vi "主画面.vi"() -> ()   [LabVIEW 2016]
uses:
  <vilib>/Utility/sysdir.llb/System Directory Type.ctl
  data/FreeMem.dll
  API/update/update/update.lvlib
panel:
  out "SN":string="系列号"
  in  "关于":bool
  in  "全屏":T1
  out "站点名称":string="站点名称"
  out "时间显示":string="2017-05-09 10:50:42"
  in  "主画面菜单":enum32{"首页", "数据查询", "运维调试", "系统设置"}(xcontrol)
  # "ESTD-XP一体化水质自动监测系统"
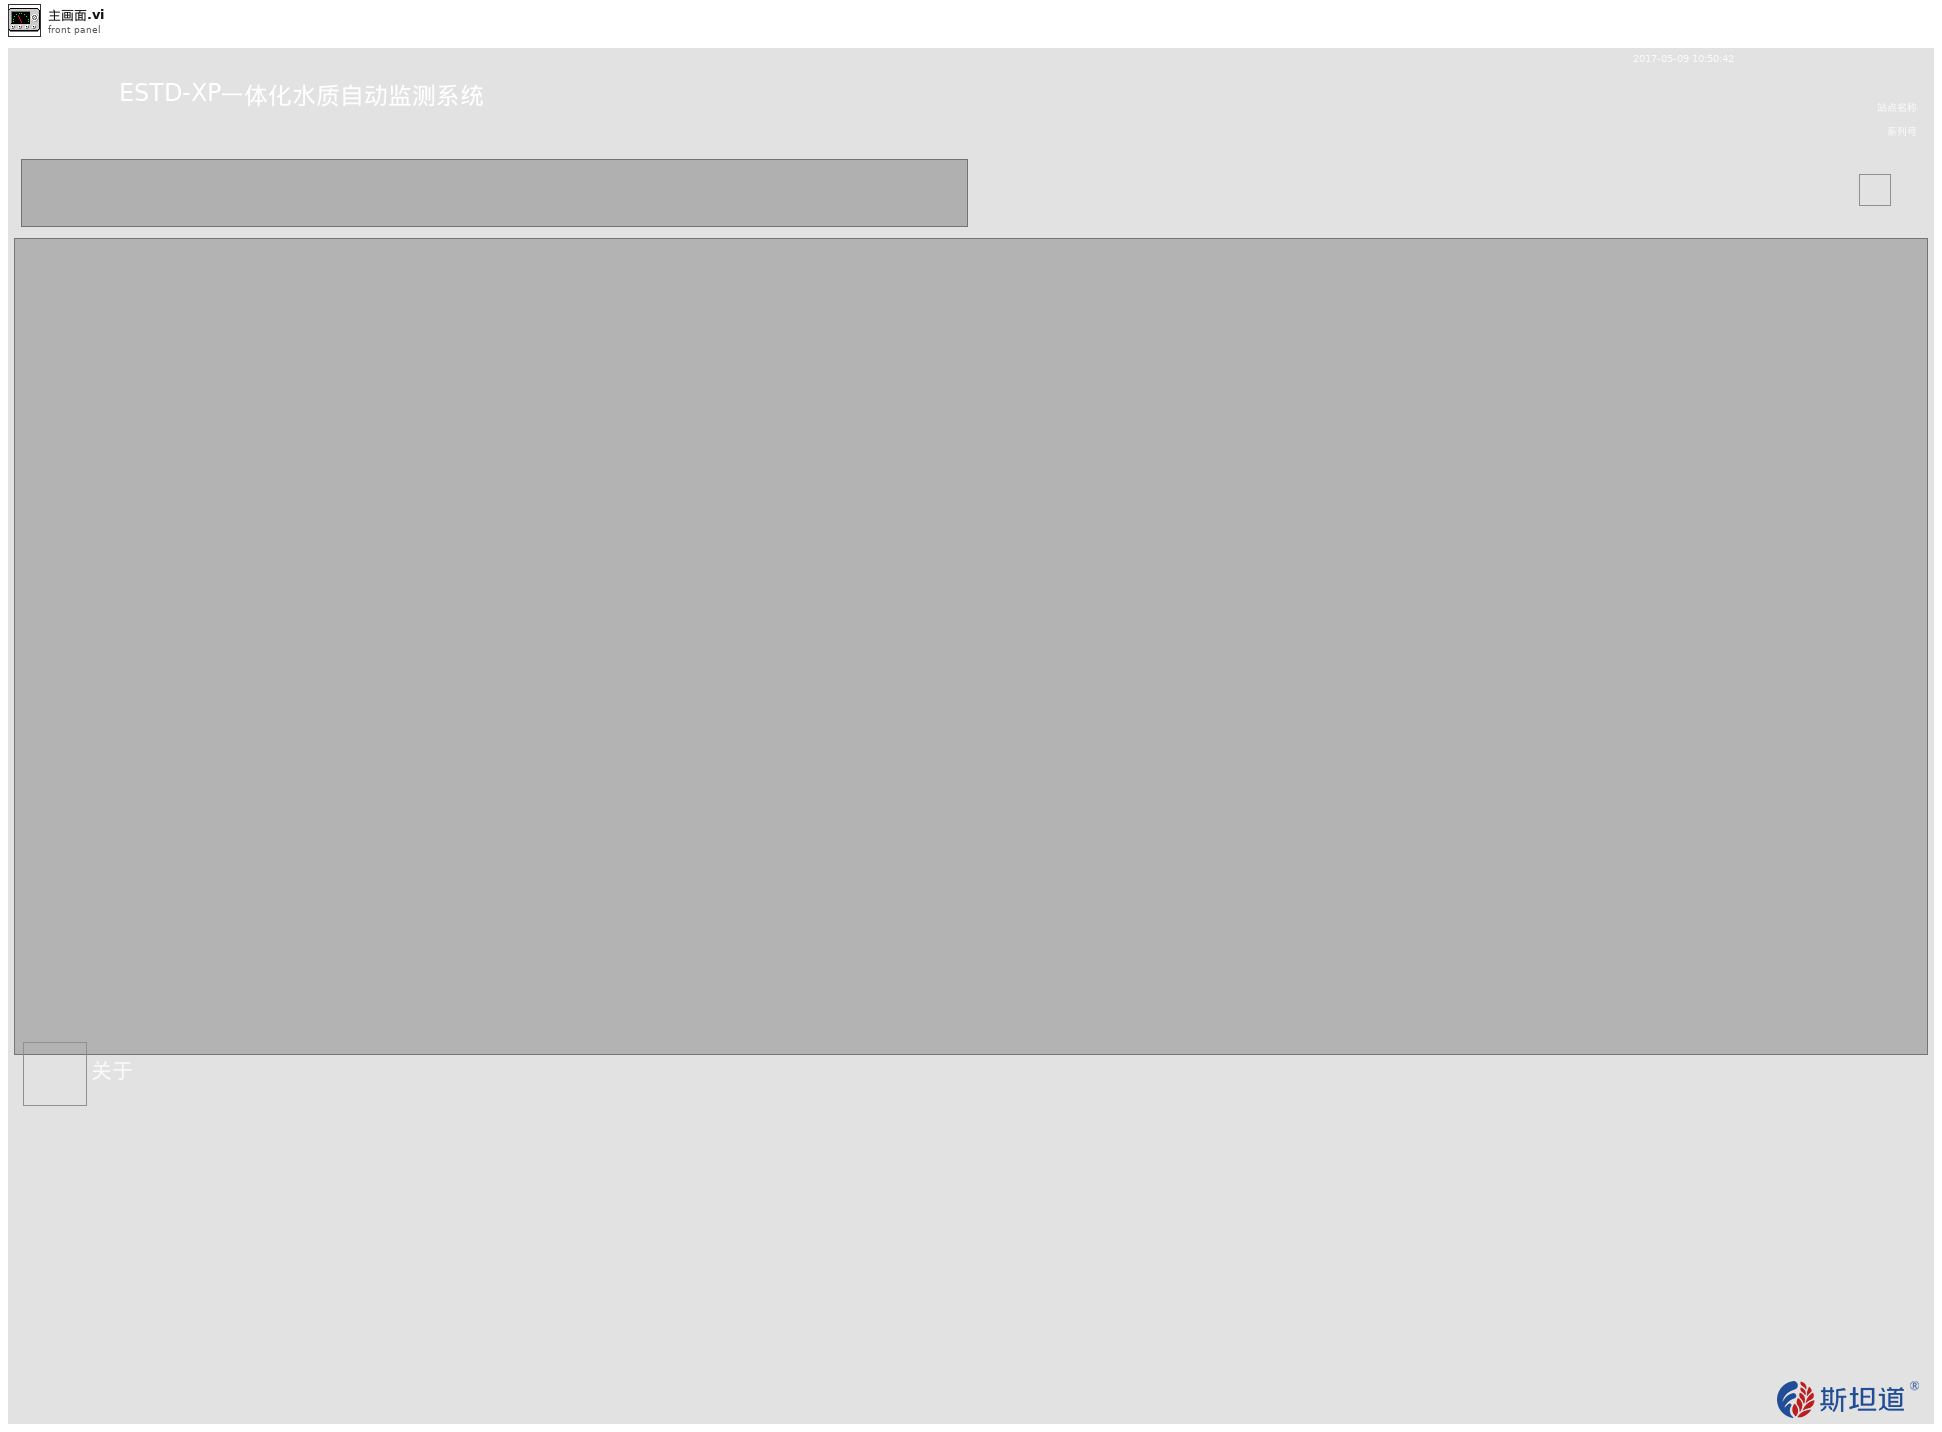
[diagram p1: front panel]
types:
  T1 = typedef "全屏按钮.ctl" = bool
  T2 = typedef "System Directory Type.ctl" = i32
  T3 = cluster{"时间标识":timestamp, "设备":string, "日志信息":string, "流程参数":string}
  T4 = enum32{"Bad", "Idle", "Run top level", "Running"}
  T5 = cluster{"host":string, "user":string, "password":string, "远端地址":string}
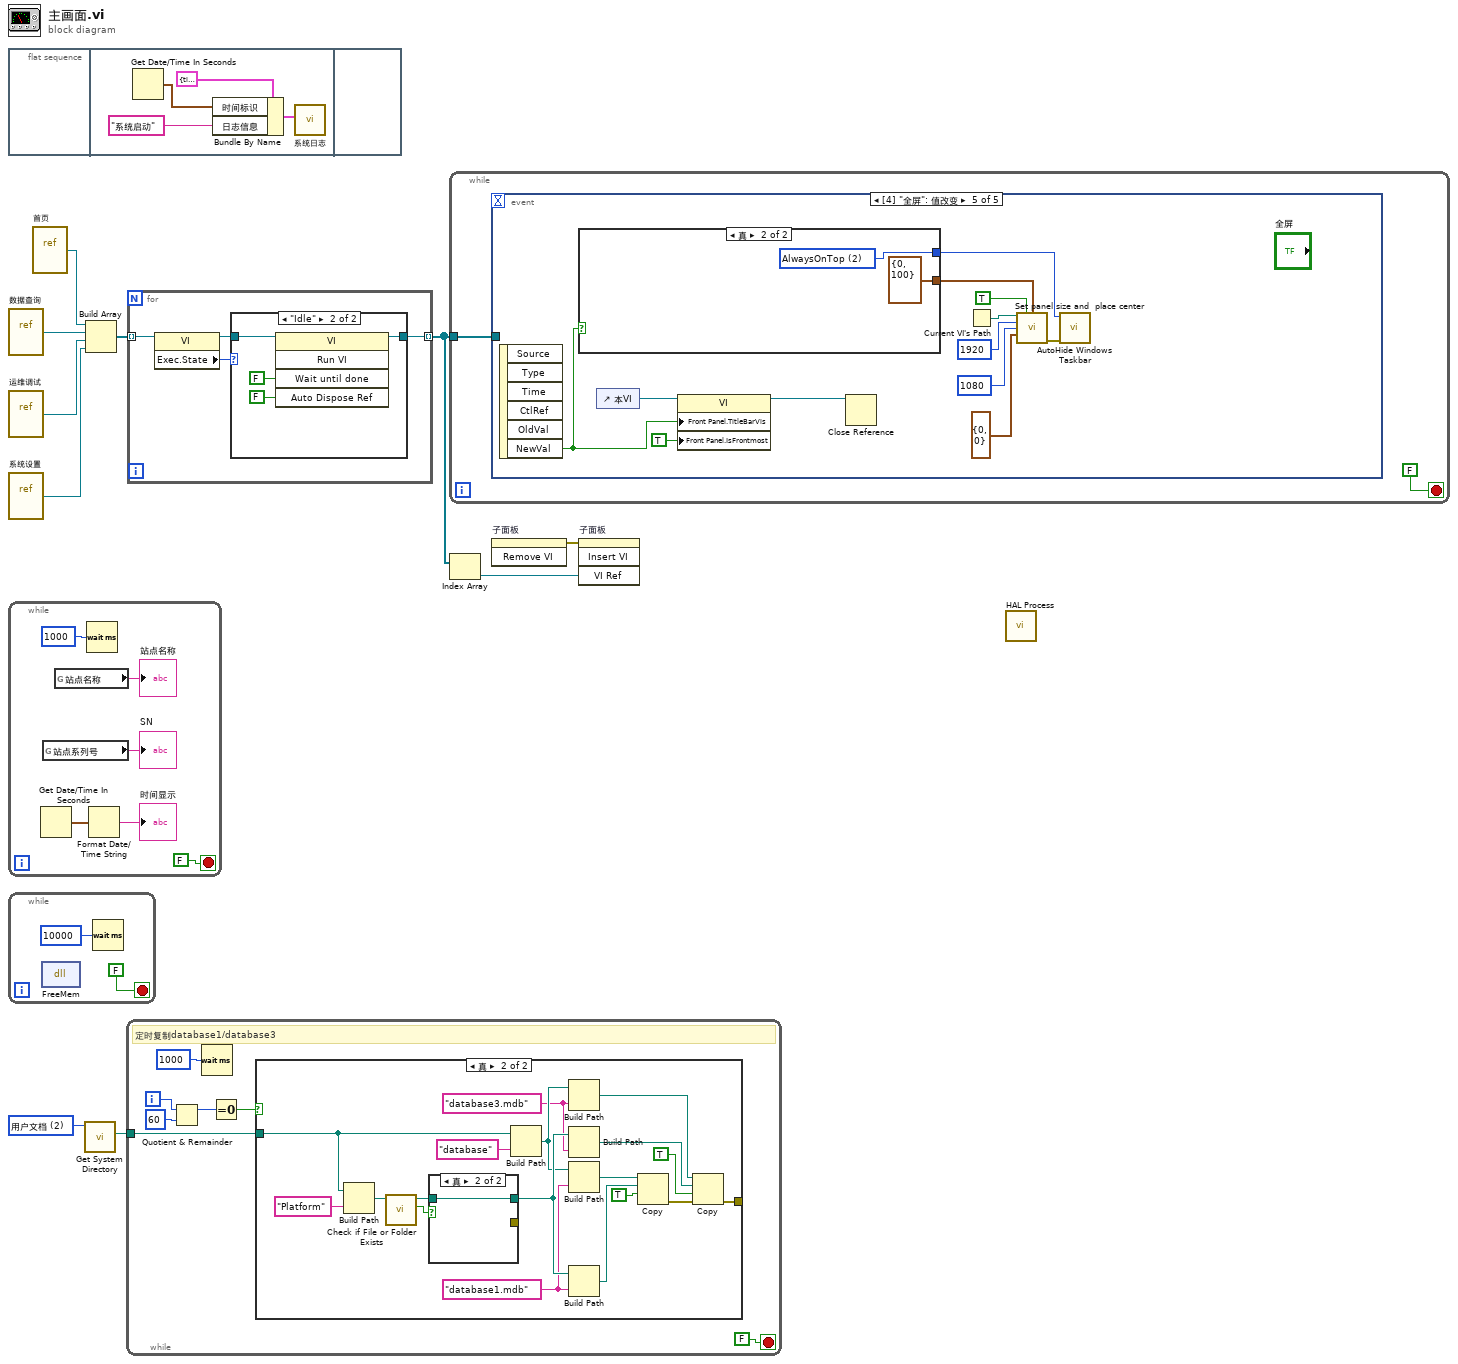
[diagram p0: block diagram]
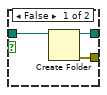
[diagram p3: hidden frame]
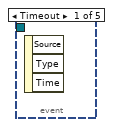
[diagram p5: hidden frame]
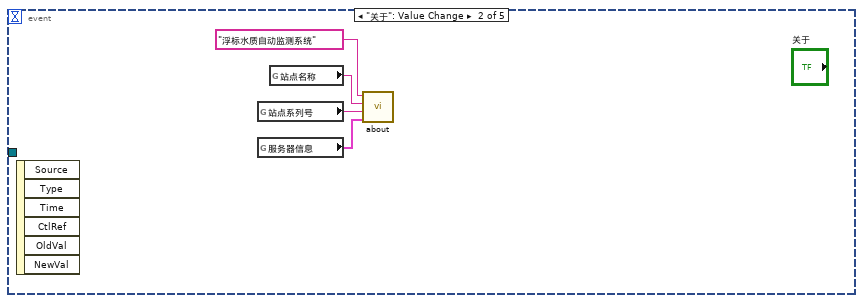
[diagram p6: hidden frame]
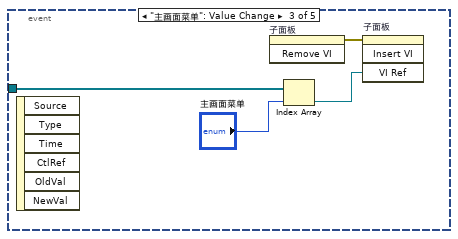
[diagram p7: hidden frame]
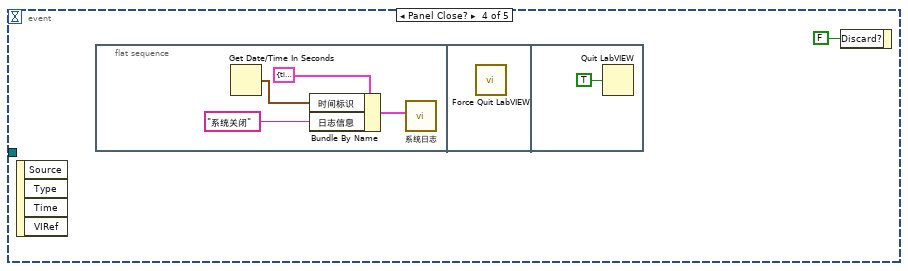
[diagram p8: hidden frame]
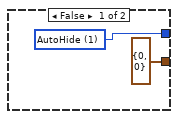
[diagram p9: hidden frame]
diagram:
  w2 = T2 2 items=["用户目录"=0, "用户桌面"=1, "用户文档"=2, "用户应用程序数据"=3, "用户设置"=4, "用户临时目录"=5, "公共文档"=6, "公共应用程序数据"=7, "公共设置"=8, "公共缓存"=13, "系统核心库"=9, "系统安装库"=10, "应用程序文件"=11, "启动盘根目录"=12] ("system directory type")
  n1 = flat-sequence {
    frame #0 {
    }
    frame #1 {
      n2 = Get Date/Time In Seconds() -> (seconds since 1Jan1904=w12:timestamp)
      n3 = Bundle By Name(cluster=T3 {"时间标识"=timestamp(0 s since 1904-01-01), "设备"="系统", "日志信息"="", "流程参数"=""} ("data in"), "时间标识"=w12, "日志信息"="系统启动") -> (w13:T3)
      n4 = call "系统日志.vi"("data in"=w13) -> ()  [unwired: 11 in]
    }
    frame #2 {
    }
  }
  n5 = vi-ref "数据查询.vi"() -> (w6:refnum<vi>)
  n6 = vi-ref "运维调试.vi"() -> (w5:refnum<vi>)
  n7 = vi-ref "系统设置.vi"() -> (w4:refnum<vi>)
  n8 = while {
    stop <- FALSE stop-if-true
    n9 = Get Date/Time In Seconds() -> (seconds since 1Jan1904=w17:timestamp)
    n10 = global read "系统设置全局变量.vi" "站点系列号"() -> (→"SN":string)
    n11 = global read "系统设置全局变量.vi" "站点名称"() -> (→"站点名称":string)
    n12 = Wait (ms)(milliseconds to wait=u32 1000 ("等待时间（毫秒）")) -> ()  [unwired: 1 out]
    n13 = Format Date/Time String(seconds (now)=w17) -> (date/time string=→"时间显示":string)  [unwired: 2 in]
  }
  n14 = while {
    stop <- FALSE stop-if-true
    n15 = dll-call lib="PTH2Fabs DGIT Source Code浮船模板source codedataFreeMem.dll" fn="FreeMem"() -> ()  [unwired: 4 in, 2 out]
    n16 = Wait (ms)(milliseconds to wait=u32 10000 ("等待时间（毫秒）")) -> ()  [unwired: 1 out]
  }
  n17 = vi-ref "首页.vi"() -> (w7:refnum<vi>)
  n18 = call <vilib>:"Get System Directory.vi"("system directory type"=w2) -> ("system directory"=w1:path)  [unwired: 10 in]
  n19 = Build Array(w7, w6, w5, w4) -> (w3:refnum<vi>[])
  n20 = while {
    tunnel: w1 -> [w23]
    i -> [w27]
    stop <- FALSE stop-if-true
    # "定时复制database1/database3"
    n21 = Quotient & Remainder(x=w27, y=60) -> (x-y*floor(x/y)=w25:i32)  [unwired: 1 out]
    n22 = Wait (ms)(milliseconds to wait=u32 1000 ("等待时间（毫秒）")) -> ()  [unwired: 1 out]
    n23 = Equal To 0?(x=w25) -> (x = 0?=w24:bool)
    n24 = case shown="真" w24 {
      tunnel: w23 -> [_ w37]
      tunnel: [_ w33] -> _
      frame False {
      }
      frame True {
        w31 = "database1.mdb" ("名称或相对路径")
        w32 = "database3.mdb" ("名称或相对路径")
        n25 = Build Path(base path=w37, name or relative path="Platform" ("名称或相对路径")) -> (appended path=w44:path)
        n26 = call <vilib>:"Check if File or Folder Exists.vi"("path"=w44) -> ("file or folder exists?"=w43:bool, "dup path"=w42:path)  [unwired: 8 in, 1 out]
        n27 = case shown="真" w43 {
          tunnel: [w49 w51] -> w39
          tunnel: w42 -> [w50 w51]
          tunnel: [w48 _] -> _
          frame False {
            n28 = Create Folder(path (use dialog)=w50) -> (created path=w49:path, error out=w48:errorcluster)  [unwired: 2 in, 1 out]
          }
          frame True {
          }
        }
        n29 = Build Path(base path=w37, name or relative path="database" ("名称或相对路径")) -> (appended path=w35:path)
        n30 = Build Path(base path=w35, name or relative path=w32) -> (appended path=w34:path)
        n31 = Build Path(base path=w39, name or relative path=w32) -> (appended path=w38:path)
        n32 = Build Path(base path=w35, name or relative path=w31) -> (appended path=w36:path)
        n33 = Build Path(base path=w39, name or relative path=w31) -> (appended path=w41:path)
        n34 = Copy(9:TRUE ("覆盖(F)"), 10:w41, 11:w36) -> (0:w40:errorcluster)  [unwired: 2 in, 2 out]
        n35 = Copy(8:w40, 9:TRUE ("覆盖(F)"), 10:w38, 11:w34) -> (0:w33:errorcluster)  [unwired: 1 in, 2 out]
      }
    }
  }
  n36 = for {
    tunnel: w3 -> [w55] mode=indexing
    tunnel: [w52] -> w9 mode=indexing
    n37 = property class="VI"(reference=w55) -> (reference out=w53:refnum<vi>, "Exec.State"=w54:T4)  [unwired: 1 in, 1 out]
    n38 = case shown="\"Idle\"" w54 {
      tunnel: w53 -> [w56 w58]
      tunnel: [w56 w57] -> w52
      frame "Bad", Default {
      }
      frame "Idle" {
        n39 = invoke class="VI" method="Run VI"(reference=w58, "Wait until done"=FALSE ("结束前等待"), "Auto Dispose Ref"=FALSE ("自动销毁引用")) -> (reference out=w57:refnum<vi>)  [unwired: 2 in, 4 out]
      }
    }
  }
  n40 = while {
    tunnel: w9 -> [w61]
    stop <- FALSE stop-if-true
    n41 = event shown="[4] \"全屏\": 值改变" {
      selector: _ -> [_ _ _ _ _]
      dyn-events: _ -> [_ _ _ _ _]
      timeout: _ -> [_ _ _ _ _]
      tunnel: w61 -> [_ _ w69 _ _]
      event Timeout {
        n42 = event-data() -> ()  [unwired: 1 in, 3 out]
      }
      event "关于": Value Change {
        n43 = event-data() -> ()  [unwired: 1 in, 6 out]
        n44 = global read "系统设置全局变量.vi" "站点系列号"() -> (w65:string)
        n45 = global read "系统设置全局变量.vi" "服务器信息"() -> (w63:T5)
        n46 = global read "系统设置全局变量.vi" "站点名称"() -> (w64:string)
        n47 = call "about.vi"("服务器信息"=w63, "SN输入"=w65, "站点名称输入"=w64, "应用程序名称输入"="浮标水质自动监测系统") -> ()  [unwired: 8 in]
      }
      event "主画面菜单": Value Change {
        n48 = event-data() -> ()  [unwired: 1 in, 6 out]
        n49 = invoke on="子面板" class="SubPnl" method="Remove VI"() -> (error out=w67:errorcluster)  [unwired: 3 in, 2 out]
        n50 = Index Array(array=w69, index="主画面菜单") -> (element=w68:refnum<vi>)
        n51 = invoke on="子面板" class="SubPnl" method="Insert VI"(error in=w67, "VI Ref"=w68) -> ()  [unwired: 2 in, 4 out]
      }
      event Panel Close? {
        n52 = event-data() -> ()  [unwired: 1 in, 4 out]
        n53 = flat-sequence {
          frame #0 {
            n54 = Get Date/Time In Seconds() -> (seconds since 1Jan1904=w74:timestamp)
            n55 = Bundle By Name(cluster=T3 {"时间标识"=timestamp(0 s since 1904-01-01), "设备"="系统", "日志信息"="", "流程参数"=""} ("data in"), "时间标识"=w74, "日志信息"="系统关闭") -> (w73:T3)
            n56 = call "系统日志.vi"("data in"=w73) -> ()  [unwired: 11 in]
          }
          frame #1 {
            n57 = call "Force Quit LabVIEW.vi"() -> ()  [unwired: 10 in, 2 out]
          }
          frame #2 {
            n58 = Quit LabVIEW(quit? (T)=TRUE ("退出？(T)")) -> ()
          }
        }
        n59 = event-data("Discard?"=FALSE ("放弃？")) -> ()  [unwired: 1 in, 1 out]
      }
      event Value Change {
        n60 = event-data() -> ("NewVal"=w83:T1)  [unwired: 1 in, 5 out]
        n61 = case shown="真" w83 {
          tunnel: [cluster{"Horizontal":i16, "Vertical":i16} {"Horizontal"=0, "Vertical"=0} ("FP.WinOrigin in(H & V)") cluster{"Horizontal":i16, "Vertical":i16} {"Horizontal"=0, "Vertical"=100} ("FP.WinOrigin in(H & V)")] -> w81
          tunnel: [w89 w91] -> w79
          frame False {
            w89 = u8 1 items=["AutoHide"=1, "AlwaysOnTop"=2] ("Operation")
          }
          frame True {
            w91 = u8 2 items=["AutoHide"=1, "AlwaysOnTop"=2] ("Operation")
          }
        }
        n62 = control-ref of="本VI"() -> (w88:refnum<vi>)
        n63 = property class="VI"(reference=w88, "Front Panel.TitleBarVis"=w83, "Front Panel.IsFrontmost"=TRUE ("前面板窗口:在最前")) -> (reference out=w84:refnum<vi>)  [unwired: 1 in, 1 out]
        n64 = Close Reference(reference=w84) -> ()  [unwired: 1 in, 1 out]
        n65 = Current VI's Path() -> (path=w87:path)
        n66 = call "Set panel size and  place center.vi"("Path"=w87, "Close Reference (false)"=TRUE, "FP.WinOrigin in(H & V)"=w81, "Panel Width"=1920, "Panel Height"=1080, "FP.Origin in(H & V)"=cluster{"Horizontal":i16, "Vertical":i16} {"Horizontal"=0, "Vertical"=0}) -> ("error out"=w80:errorcluster)  [unwired: 8 in, 1 out]
        n67 = call "AutoHide Windows Taskbar.vi"("error in (no error)"=w80, "Operation"=w79) -> ()  [unwired: 5 in, 1 out]
      }
    }
  }
  n68 = Index Array(array=w9) -> (element=w8:refnum<vi>)  [unwired: 1 in]
  n69 = invoke on="子面板" class="SubPnl" method="Remove VI"() -> (error out=w10:errorcluster)  [unwired: 3 in, 2 out]
  n70 = invoke on="子面板" class="SubPnl" method="Insert VI"(error in=w10, "VI Ref"=w8) -> ()  [unwired: 2 in, 4 out]
  n71 = call "HAL Process.vi"() -> ()  [unwired: 12 in]
